vi "GetBarcode 1DResultValue.vi"(8 "error in (no error)":errorcluster, 9 "data":T1(array[cluster]), 11 "Analysis_Barcode 1D_Parameter":T2={"Barcode Search Options"={"Min Bar Width"=0.0, "Min Edge Strength"=0.0, "Min Bars"=0.0, "Skip Location Search?"=FALSE}, "Barcode Types To Search"=[enum."EAN 13", enum."Code 128", enum."Code 39"], "Barcode Grading Options"={"Calculate Grading Report"=FALSE, "Scan Width "=0.0}, "Number of Matches Requested"=1, "ROI"={"Global Rectangle"=[], "Contours"=[]}}) -> (0 "error out":errorcluster, 3 "ResultValues":string[](array[string]))   [LabVIEW 2019]
uses:
  Controls/Barcode 1D/Analysis_Barcode 1D_Parameter.ctl
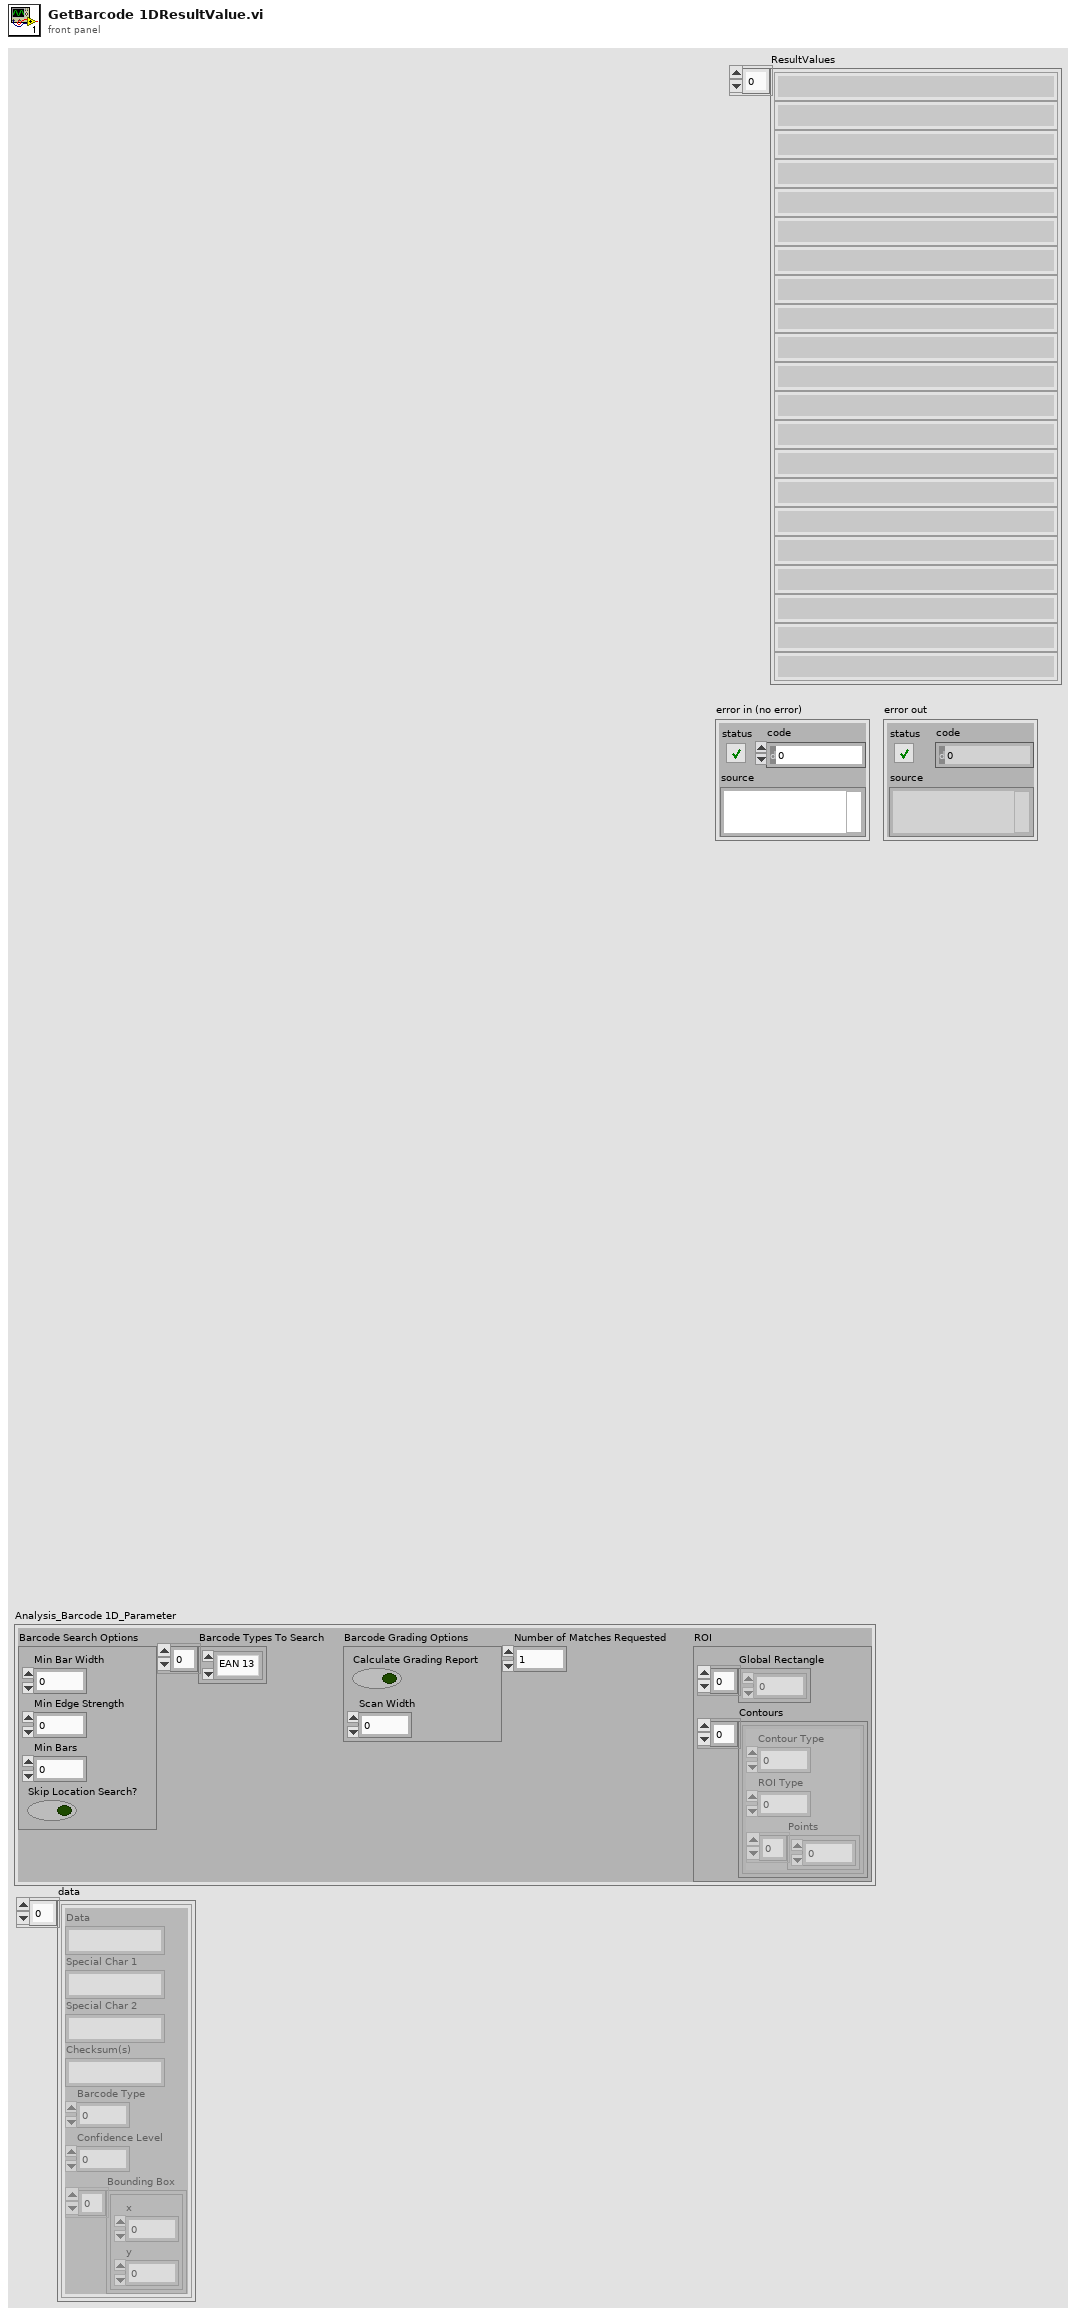
[diagram p1: front panel]
types:
  T1 = cluster{"Data":string, "Special Char 1":string, "Special Char 2":string, "Checksum(s)":string, "Barcode Type":u32, "Confidence Level":sgl, "Bounding Box":cluster{"x":sgl, "y":sgl}[]}[]
  T2 = typedef "Analysis_Barcode 1D_Parameter.ctl" = cluster{"Barcode Search Options":cluster{"Min Bar Width":dbl, "Min Edge Strength":dbl, "Min Bars":dbl, "Skip Location Search?":bool}, "Barcode Types To Search":enum16{"Reserved", "Codabar", "Code 39", "Code 93", "Code 128", "EAN 8", "EAN 13", "Interleaved 2 of 5", "MSI", "UPCA", "Pharmacode", "RSS Limited"}[], "Barcode Grading Options":cluster{"Calculate Grading Report":bool, "Scan Width ":dbl}, "Number of Matches Requested":i32, "ROI":cluster{"Global Rectangle":i32[], "Contours":cluster{"Contour Type":u32, "ROI Type":u32, "Points":i32[]}[]}}
  T3 = cluster{"Data":string, "Special Char 1":string, "Special Char 2":string, "Checksum(s)":string, "Barcode Type":u32, "Confidence Level":sgl, "Bounding Box":cluster{"x":sgl, "y":sgl}[]}
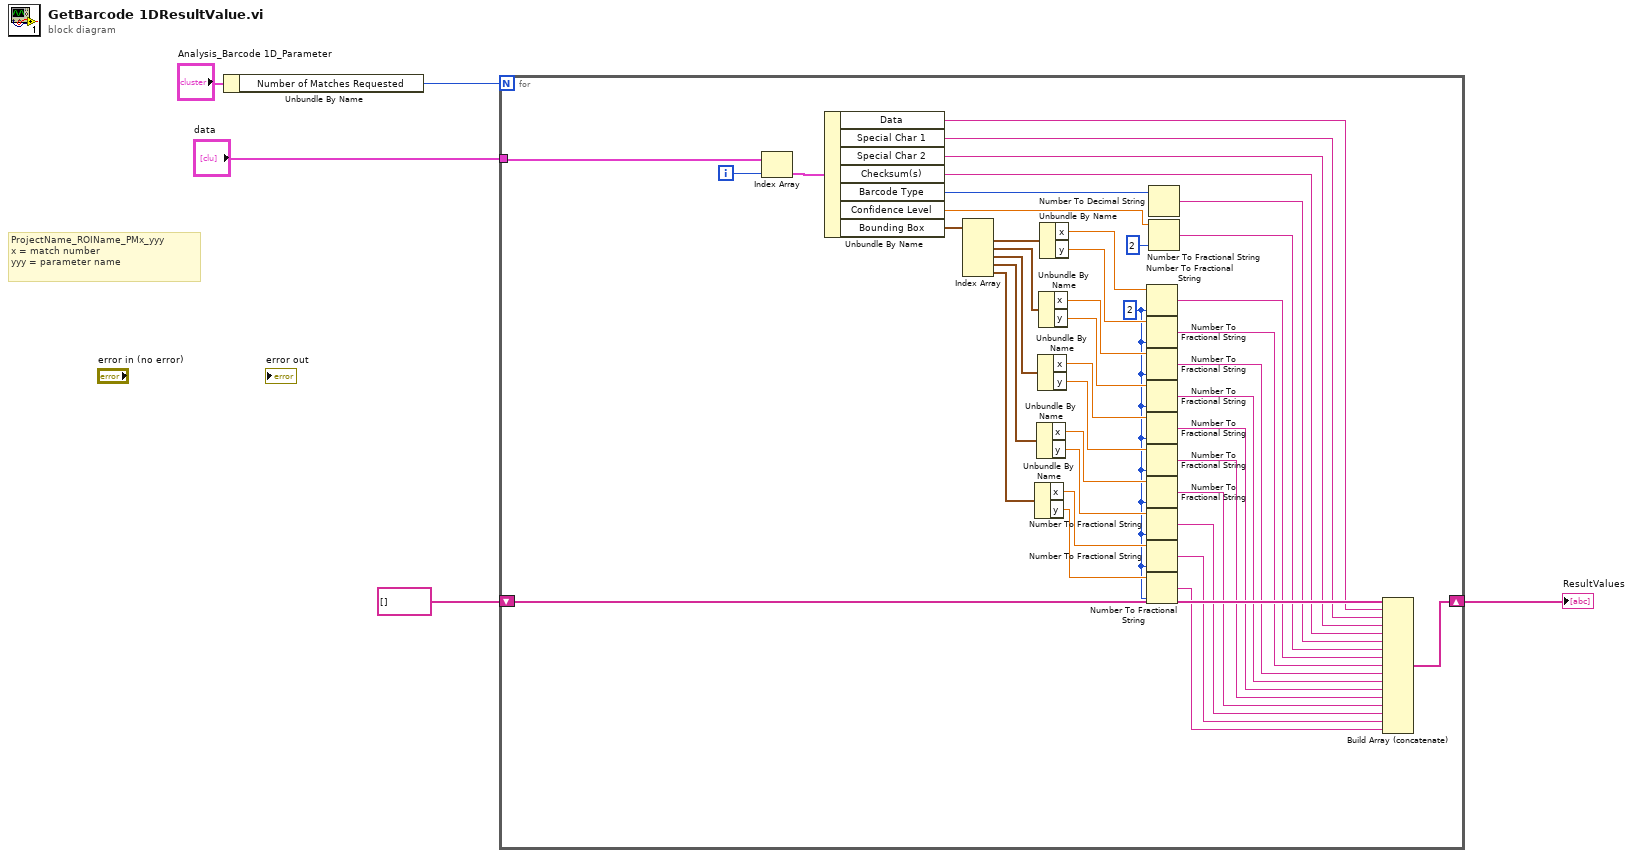
[diagram p0: block diagram]
diagram:
  # "ProjectName_ROIName_PMx_yyy\nx = match number\nyyy = parameter name"
  n1 = Unbundle By Name("Analysis_Barcode 1D_Parameter") -> ("Number of Matches Requested"=w2:i32)
  n2 = for {
    N: w2 -> [_]
    shift-right: [w44] -> w4
    shift-left: string[] [] -> [w45]
    tunnel: "data" -> [w6]
    i -> [w43]
    w17 = i16 2 ("precision (6)")
    n3 = Index Array(array=w6, index=w43) -> (element=w46:T3)
    n4 = Unbundle By Name(w46) -> ("Data"=w42:string, "Special Char 1"=w41:string, "Special Char 2"=w40:string, "Checksum(s)"=w39:string, "Barcode Type"=w38:u32, "Confidence Level"=w35:sgl, "Bounding Box"=w33:cluster{"x":sgl, "y":sgl}[])
    n5 = Index Array(array=w33) -> (element #1=w32:cluster{"x":sgl, "y":sgl}, element #2=w31:cluster{"x":sgl, "y":sgl}, element #3=w30:cluster{"x":sgl, "y":sgl}, element #4=w29:cluster{"x":sgl, "y":sgl}, element #5=w28:cluster{"x":sgl, "y":sgl})  [unwired: 5 in]
    n6 = Unbundle By Name(w28) -> ("x"=w19:sgl, "y"=w18:sgl)
    n7 = Unbundle By Name(w29) -> ("x"=w21:sgl, "y"=w20:sgl)
    n8 = Unbundle By Name(w30) -> ("x"=w23:sgl, "y"=w22:sgl)
    n9 = Unbundle By Name(w31) -> ("x"=w25:sgl, "y"=w24:sgl)
    n10 = Unbundle By Name(w32) -> ("x"=w27:sgl, "y"=w26:sgl)
    n11 = Number To Fractional String(number=w27, precision (6)=w17) -> (F-format string=w16:string)  [unwired: 2 in]
    n12 = Number To Fractional String(number=w26, precision (6)=w17) -> (F-format string=w15:string)  [unwired: 2 in]
    n13 = Number To Fractional String(number=w25, precision (6)=w17) -> (F-format string=w14:string)  [unwired: 2 in]
    n14 = Number To Fractional String(number=w24, precision (6)=w17) -> (F-format string=w13:string)  [unwired: 2 in]
    n15 = Number To Fractional String(number=w23, precision (6)=w17) -> (F-format string=w12:string)  [unwired: 2 in]
    n16 = Number To Fractional String(number=w22, precision (6)=w17) -> (F-format string=w11:string)  [unwired: 2 in]
    n17 = Number To Fractional String(number=w21, precision (6)=w17) -> (F-format string=w10:string)  [unwired: 2 in]
    n18 = Number To Fractional String(number=w20, precision (6)=w17) -> (F-format string=w9:string)  [unwired: 2 in]
    n19 = Number To Fractional String(number=w19, precision (6)=w17) -> (F-format string=w8:string)  [unwired: 2 in]
    n20 = Number To Fractional String(number=w18, precision (6)=w17) -> (F-format string=w7:string)  [unwired: 2 in]
    n21 = Number To Decimal String(number=w38) -> (decimal integer string=w37:string)  [unwired: 1 in]
    n22 = Number To Fractional String(number=w35, precision (6)=i16 2) -> (F-format string=w34:string)  [unwired: 2 in]
    n23 = Build Array (concatenate)(w45, w42, w41, w40, w39, w37, w34, w16, w15, w14, w13, w12, w11, w10, w9, w8, w7) -> (w44:string[])
  }
  "ResultValues" <- w4
